vi "loadDataToBuffer.vi"(8 "error in (no error)":errorcluster, 11 "K2602 in":refnum<class "K2602.lvclass">) -> (0 "error out":errorcluster, 3 "K2602 out":refnum<class "K2602.lvclass">)   [LabVIEW 2009, in "Hardware.lvlib" / "Channels.lvlib" / "K2602.lvclass"]
doc: "Abstract Method.\n\nThis vi, via its implementing classes, loads the analog output data to the buffer of the device."
uses:
  K2602.lvclass
  AnalogOutput.lvclass
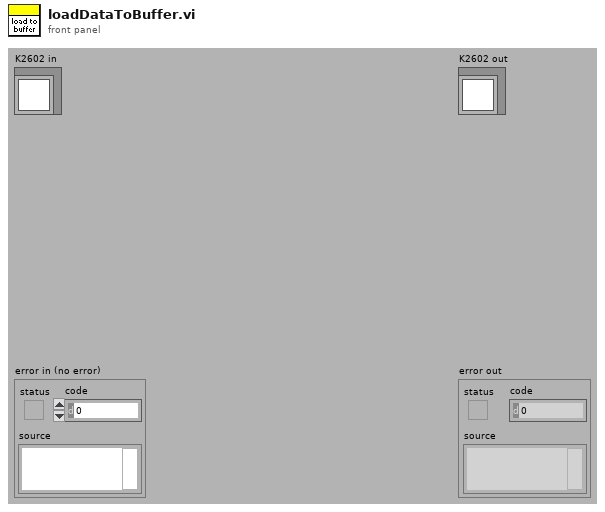
[diagram p1: front panel]
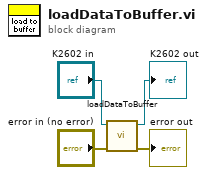
[diagram p0: block diagram]
diagram:
  n1 = call-parent "loadDataToBuffer.vi"("error in (no error)"="error in (no error)", "AnalogOutput in"="K2602 in") -> ("error out"=→"error out":errorcluster, "AnalogOutput out"=→"K2602 out":refnum<class "K2602.lvclass">)  [unwired: 8 in]
